vi "Autonomous Independent.vi"() -> ()   [LabVIEW 2016]
doc: "This VI is called when autonomous begins, and will automatically be terminated when autonomous ends. You can carry out timed or sensor driven robot movement independently without needing to return to the caller."
uses:
  <vilib>/Rock Robotics/Network Tables/NT Read String.vi
  Robot Global Data.vi
  <vilib>/Rock Robotics/WPI/Utilities/WPI_GetSetVariantRefNum.vi
  <vilib>/Rock Robotics/Network Tables/NT Write Numeric Array.vi
  2039lib.lvlib
panel:
  out "Doing Something":bool=TRUE
  # "Be sure to right-click and choose Data Operations>>Make Current Value default if you want to save the array values with the VI"
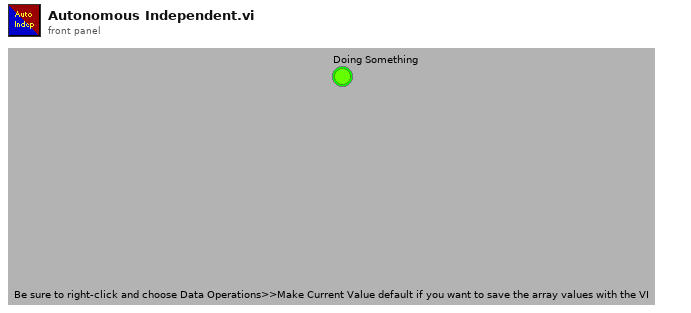
[diagram p1: front panel]
types:
  T1 = typedef "WPI_RobotDriveDevRef.ctl" = cluster{"DevStatus":errorcluster, "Motors[]":T2[], "Square Inputs":bool, "Max Output":dbl}
  T2 = typedef "WPI_MotorControlDeviceRef.ctl" = cluster{"DeviceStatus":errorcluster, "Type":T3, "PWM":cluster{"PWM Channel":T4, "DeadBand":T5}, "CAN":cluster{"Device Number":u8, "SetOutput VI Ref":variant, "GetOutput VI Ref":variant, "Enable VI Ref":variant, "Disable VI Ref":variant, "Data":variant}, "Invert":bool}
  T3 = typedef "WPI_MotorControlType.ctl" = enum16{"PWM", "CAN"}
  T4 = typedef "FPGA_DIOPWMChannel.ctl" = enum8{"PWM 0", "PWM 1", "PWM 2", "PWM 3", "PWM 4", "PWM 5", "PWM 6", "PWM 7", "PWM 8", "PWM 9", "PWM MXP 0", "PWM MXP 1", "PWM MXP 2", "PWM MXP 3", "PWM MXP 4", "PWM MXP 5", "PWM MXP 6", "PWM MXP 7", "PWM MXP 8", "PWM MXP 9", "Invalid"}
  T5 = typedef "WPI_PWMDeadband.ctl" = cluster{"Name":string, "maxPositivePwm":i32, "minPositivePwm":i32, "centerPwm":i32, "maxNegativePwm":i32, "minNegativePwm":i32, "angularRange":u16}
  T6 = typedef "WPI_ServoDeviceRef.ctl" = cluster{"DeviceStatus":errorcluster, "PWM Channel":T4, "DeadBand":T5}
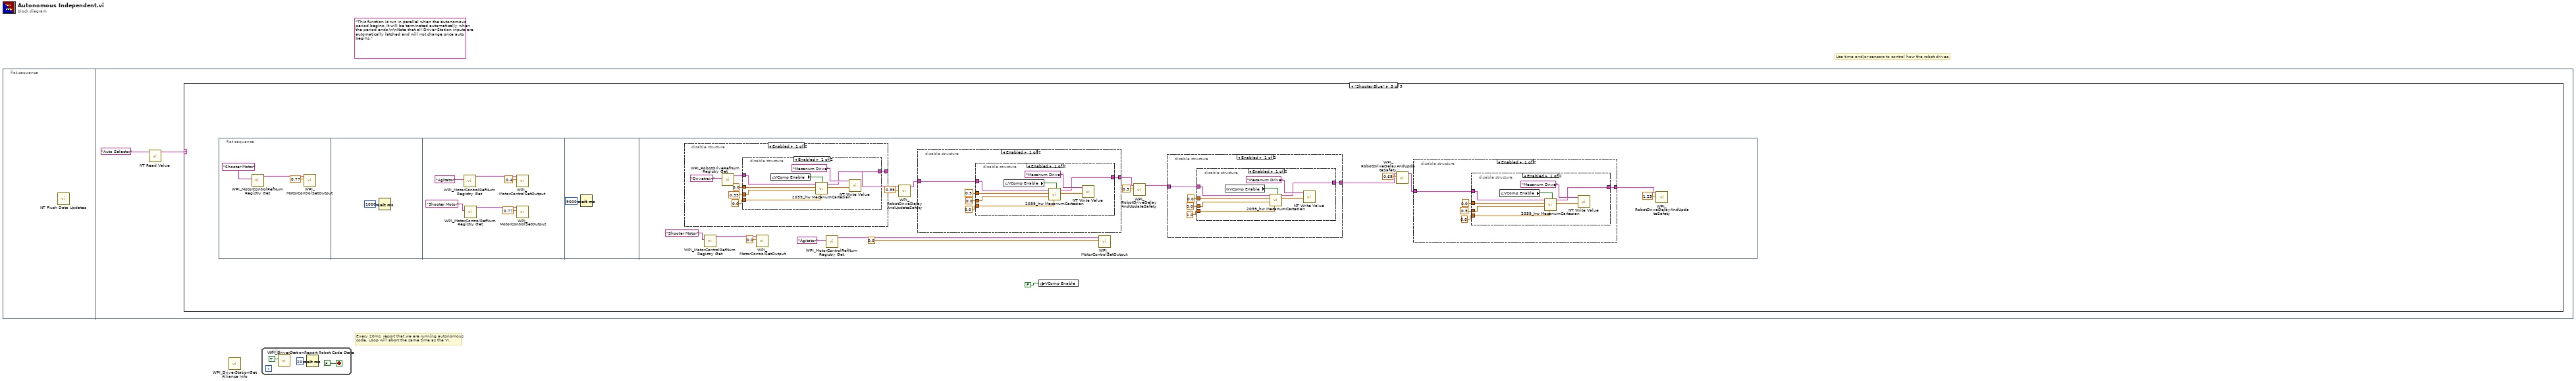
[diagram p0: block diagram]
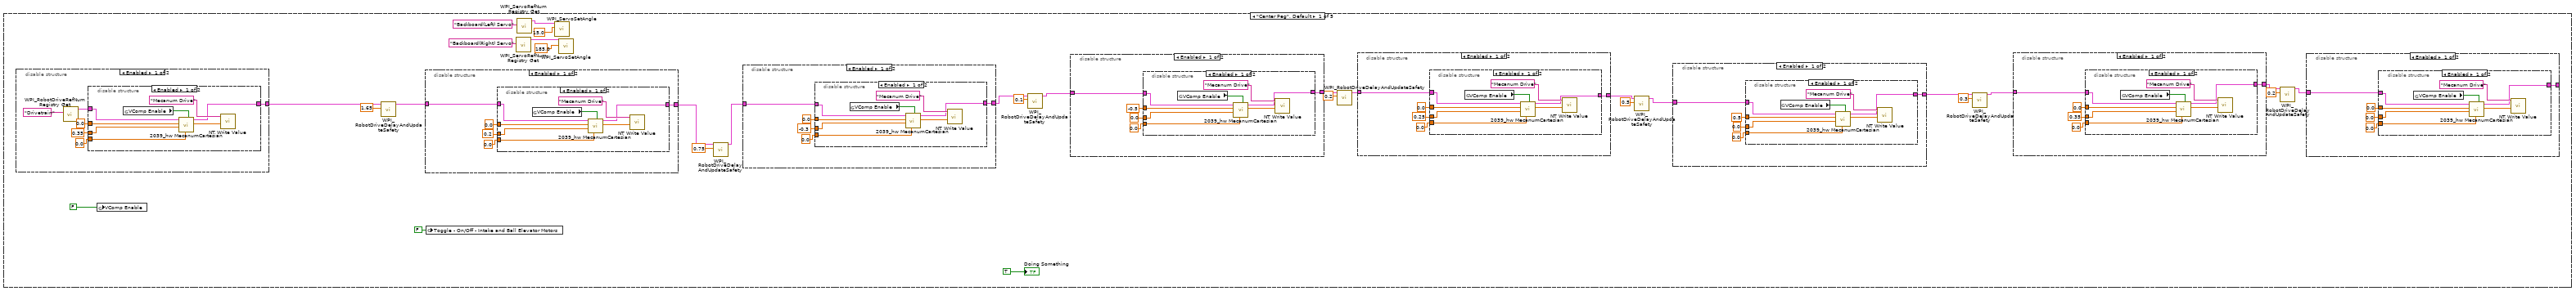
[diagram p2: hidden frame]
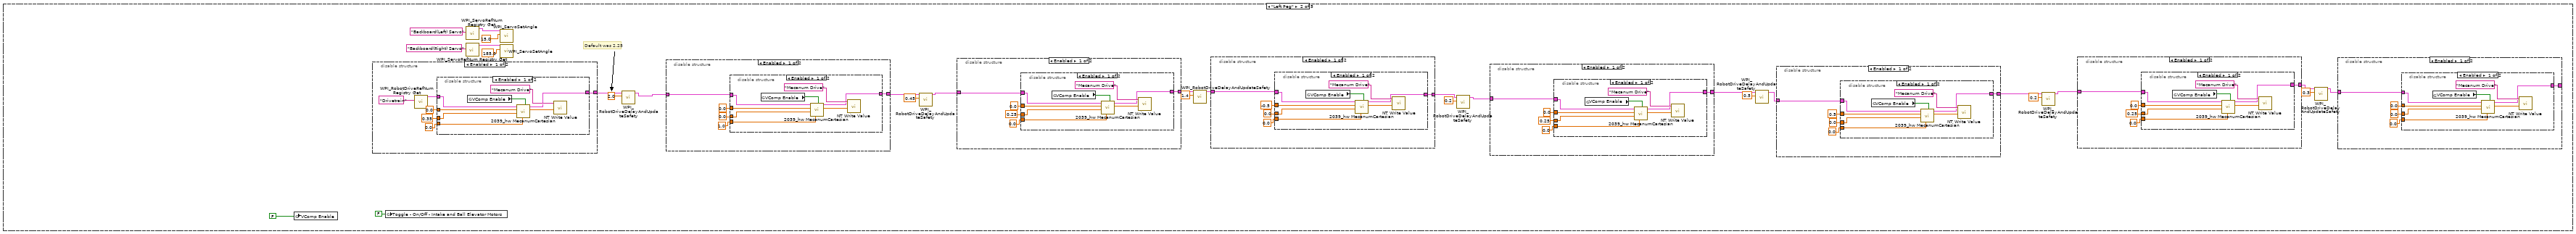
[diagram p19: hidden frame]
diagram:
  (unwired) "This function is run in parallel when the autonomous period begins. It will be terminated automatically when the period ends.\n\nNote that all Driver Station inputs are automatically latched and will not change once auto begins."
  # "Every 20ms, report that we are running autonomous\ncode. Loop will abort the same time as the VI."
  # "Use time and/or sensors to control how the robot drives."
  n1 = flat-sequence {
    frame #0 {
      n2 = call <vilib>:"NT Flush Data Updates.vi"() -> ()  [unwired: 11 in, 1 out]
    }
    frame #1 {
      n3 = call-poly <vilib>:"NT Read Value.vi"("Name"="Auto Selector") -> ("String"=w1:string)  [unwired: 9 in, 1 out]
      n4 = case shown="\"Shooter Blue\"" w1 {
        frame "Center Peg", Default {
          n5 = disable-structure shown="Enabled" {
            disable-tunnel: [w124 _] -> w31
            frame Enabled {
              n6 = call <vilib>:"WPI_RobotDriveRefNum Registry Get.vi"("refnum name"="Drivetrain") -> ("RobotDriveDevRef"=w128:T1)  [unwired: 1 in, 9 out]
              n7 = disable-structure shown="Enabled" {
                disable-tunnel: w128 -> [w137 _]
                disable-tunnel: 0.0 -> [w136 _]
                disable-tunnel: 0.0 -> [w133 _]
                disable-tunnel: 0.35 -> [w132 _]
                disable-tunnel: [w130 _] -> w124
                frame Enabled {
                  n8 = global read "Robot Global Data.vi" "VComp Enable"() -> (w131:bool)
                  n9 = call "2039_hw MecanumCartesian.vi"("VComp Scaling"=w131, "Rotation"=w136, "Y"=w132, "X"=w133, "RobotDriveDevRef"=w137) -> ("Motor Values"=w134:dbl[], "RobotDriveDevRef"=w130:T1)  [unwired: 4 in, 1 out]
                  n10 = call-poly <vilib>:"NT Write Value.vi"("Numeric Array"=w134, "Name"="Mecanum Drive") -> ()  [unwired: 9 in, 1 out]
                }
                frame Disabled {
                }
              }
            }
            frame Disabled {
            }
          }
          n11 = global write "Robot Global Data.vi" "VComp Enable"(FALSE) -> ()
          n12 = call <vilib>:"WPI_RobotDriveDelayAndUpdateSafety.vi"("Delay (s)"=1.65, "RobotDriveDevRef"=w31) -> ("RobotDriveDevRef 2"=w5:T1)  [unwired: 8 in, 1 out]
          n13 = disable-structure shown="Enabled" {
            disable-tunnel: [w34 _] -> w7
            disable-tunnel: w5 -> [w33 _]
            frame Enabled {
              n14 = disable-structure shown="Enabled" {
                disable-tunnel: 0.0 -> [w45 _]
                disable-tunnel: 0.0 -> [w42 _]
                disable-tunnel: 0.2 -> [w41 _]
                disable-tunnel: [w39 _] -> w34
                disable-tunnel: w33 -> [w38 _]
                frame Enabled {
                  n15 = global read "Robot Global Data.vi" "VComp Enable"() -> (w40:bool)
                  n16 = call "2039_hw MecanumCartesian.vi"("VComp Scaling"=w40, "Rotation"=w45, "Y"=w41, "X"=w42, "RobotDriveDevRef"=w38) -> ("Motor Values"=w43:dbl[], "RobotDriveDevRef"=w39:T1)  [unwired: 4 in, 1 out]
                  n17 = call-poly <vilib>:"NT Write Value.vi"("Numeric Array"=w43, "Name"="Mecanum Drive") -> ()  [unwired: 9 in, 1 out]
                }
                frame Disabled {
                }
              }
            }
            frame Disabled {
            }
          }
          n18 = global write "Robot Global Data.vi" "Toggle - On/Off - Intake and Ball Elevator Motors"(FALSE ("Toggle - On/Off - Intake and Ball Elevator Motors")) -> ()
          n19 = call <vilib>:"WPI_ServoRefNum Registry Get.vi"("refnum name"="Backboard(Right) Servo") -> ("ServoDeviceRef"=w17:T6)  [unwired: 9 in, 1 out]
          n20 = call <vilib>:"WPI_ServoRefNum Registry Get.vi"("refnum name"="Backboard(Left) Servo") -> ("ServoDeviceRef"=w18:T6)  [unwired: 9 in, 1 out]
          n21 = call <vilib>:"WPI_ServoSetAngle.vi"("Angle"=15.0 ("f"), "ServoDeviceRef"=w18) -> ()  [unwired: 8 in, 2 out]
          n22 = call <vilib>:"WPI_ServoSetAngle.vi"("Angle"=185.0 ("f"), "ServoDeviceRef"=w17) -> ()  [unwired: 8 in, 2 out]
          n23 = call <vilib>:"WPI_RobotDriveDelayAndUpdateSafety.vi"("Delay (s)"=0.75, "RobotDriveDevRef"=w7) -> ("RobotDriveDevRef 2"=w4:T1)  [unwired: 8 in, 1 out]
          n24 = disable-structure shown="Enabled" {
            disable-tunnel: w4 -> [w47 _]
            disable-tunnel: [w46 _] -> w11
            frame Enabled {
              n25 = disable-structure shown="Enabled" {
                disable-tunnel: w47 -> [w58 _]
                disable-tunnel: 0.0 -> [w57 _]
                disable-tunnel: 0.0 -> [w54 _]
                disable-tunnel: -0.3 -> [w53 _]
                disable-tunnel: [w51 _] -> w46
                frame Enabled {
                  n26 = global read "Robot Global Data.vi" "VComp Enable"() -> (w52:bool)
                  n27 = call "2039_hw MecanumCartesian.vi"("VComp Scaling"=w52, "Rotation"=w57, "Y"=w53, "X"=w54, "RobotDriveDevRef"=w58) -> ("Motor Values"=w55:dbl[], "RobotDriveDevRef"=w51:T1)  [unwired: 4 in, 1 out]
                  n28 = call-poly <vilib>:"NT Write Value.vi"("Numeric Array"=w55, "Name"="Mecanum Drive") -> ()  [unwired: 9 in, 1 out]
                }
                frame Disabled {
                }
              }
            }
            frame Disabled {
            }
          }
          n29 = call <vilib>:"WPI_RobotDriveDelayAndUpdateSafety.vi"("Delay (s)"=0.1, "RobotDriveDevRef"=w11) -> ("RobotDriveDevRef 2"=w10:T1)  [unwired: 8 in, 1 out]
          n30 = disable-structure shown="Enabled" {
            disable-tunnel: w10 -> [w112 _]
            disable-tunnel: [w111 _] -> w29
            frame Enabled {
              n31 = disable-structure shown="Enabled" {
                disable-tunnel: w112 -> [w123 _]
                disable-tunnel: 0.0 -> [w122 _]
                disable-tunnel: -0.5 -> [w119 _]
                disable-tunnel: 0.0 -> [w118 _]
                disable-tunnel: [w116 _] -> w111
                frame Enabled {
                  n32 = global read "Robot Global Data.vi" "VComp Enable"() -> (w117:bool)
                  n33 = call "2039_hw MecanumCartesian.vi"("VComp Scaling"=w117, "Rotation"=w122, "Y"=w118, "X"=w119, "RobotDriveDevRef"=w123) -> ("Motor Values"=w120:dbl[], "RobotDriveDevRef"=w116:T1)  [unwired: 4 in, 1 out]
                  n34 = call-poly <vilib>:"NT Write Value.vi"("Numeric Array"=w120, "Name"="Mecanum Drive") -> ()  [unwired: 9 in, 1 out]
                }
                frame Disabled {
                }
              }
            }
            frame Disabled {
            }
          }
          n35 = call <vilib>:"WPI_RobotDriveDelayAndUpdateSafety.vi"("Delay (s)"=0.2, "RobotDriveDevRef"=w29) -> ("RobotDriveDevRef 2"=w28:T1)  [unwired: 8 in, 1 out]
          n36 = disable-structure shown="Enabled" {
            disable-tunnel: w28 -> [w99 _]
            disable-tunnel: [w98 _] -> w26
            frame Enabled {
              n37 = disable-structure shown="Enabled" {
                disable-tunnel: w99 -> [w110 _]
                disable-tunnel: 0.0 -> [w109 _]
                disable-tunnel: 0.0 -> [w106 _]
                disable-tunnel: 0.25 -> [w105 _]
                disable-tunnel: [w103 _] -> w98
                frame Enabled {
                  n38 = global read "Robot Global Data.vi" "VComp Enable"() -> (w104:bool)
                  n39 = call "2039_hw MecanumCartesian.vi"("VComp Scaling"=w104, "Rotation"=w109, "Y"=w105, "X"=w106, "RobotDriveDevRef"=w110) -> ("Motor Values"=w107:dbl[], "RobotDriveDevRef"=w103:T1)  [unwired: 4 in, 1 out]
                  n40 = call-poly <vilib>:"NT Write Value.vi"("Numeric Array"=w107, "Name"="Mecanum Drive") -> ()  [unwired: 9 in, 1 out]
                }
                frame Disabled {
                }
              }
            }
            frame Disabled {
            }
          }
          n41 = call <vilib>:"WPI_RobotDriveDelayAndUpdateSafety.vi"("Delay (s)"=0.5, "RobotDriveDevRef"=w26) -> ("RobotDriveDevRef 2"=w25:T1)  [unwired: 8 in, 1 out]
          n42 = disable-structure shown="Enabled" {
            disable-tunnel: w25 -> [w86 _]
            disable-tunnel: [w85 _] -> w23
            frame Enabled {
              n43 = disable-structure shown="Enabled" {
                disable-tunnel: w86 -> [w97 _]
                disable-tunnel: 0.0 -> [w96 _]
                disable-tunnel: 0.5 -> [w93 _]
                disable-tunnel: 0.0 -> [w92 _]
                disable-tunnel: [w90 _] -> w85
                frame Enabled {
                  n44 = global read "Robot Global Data.vi" "VComp Enable"() -> (w91:bool)
                  n45 = call "2039_hw MecanumCartesian.vi"("VComp Scaling"=w91, "Rotation"=w96, "Y"=w92, "X"=w93, "RobotDriveDevRef"=w97) -> ("Motor Values"=w94:dbl[], "RobotDriveDevRef"=w90:T1)  [unwired: 4 in, 1 out]
                  n46 = call-poly <vilib>:"NT Write Value.vi"("Numeric Array"=w94, "Name"="Mecanum Drive") -> ()  [unwired: 9 in, 1 out]
                }
                frame Disabled {
                }
              }
            }
            frame Disabled {
            }
          }
          n47 = call <vilib>:"WPI_RobotDriveDelayAndUpdateSafety.vi"("Delay (s)"=0.3, "RobotDriveDevRef"=w23) -> ("RobotDriveDevRef 2"=w21:T1)  [unwired: 8 in, 1 out]
          n48 = disable-structure shown="Enabled" {
            disable-tunnel: w21 -> [w73 _]
            disable-tunnel: [w72 _] -> w14
            frame Enabled {
              n49 = disable-structure shown="Enabled" {
                disable-tunnel: w73 -> [w84 _]
                disable-tunnel: 0.0 -> [w83 _]
                disable-tunnel: 0.0 -> [w80 _]
                disable-tunnel: 0.35 -> [w79 _]
                disable-tunnel: [w77 _] -> w72
                frame Enabled {
                  n50 = global read "Robot Global Data.vi" "VComp Enable"() -> (w78:bool)
                  n51 = call "2039_hw MecanumCartesian.vi"("VComp Scaling"=w78, "Rotation"=w83, "Y"=w79, "X"=w80, "RobotDriveDevRef"=w84) -> ("Motor Values"=w81:dbl[], "RobotDriveDevRef"=w77:T1)  [unwired: 4 in, 1 out]
                  n52 = call-poly <vilib>:"NT Write Value.vi"("Numeric Array"=w81, "Name"="Mecanum Drive") -> ()  [unwired: 9 in, 1 out]
                }
                frame Disabled {
                }
              }
            }
            frame Disabled {
            }
          }
          n53 = call <vilib>:"WPI_RobotDriveDelayAndUpdateSafety.vi"("Delay (s)"=0.2, "RobotDriveDevRef"=w14) -> ("RobotDriveDevRef 2"=w13:T1)  [unwired: 8 in, 1 out]
          n54 = disable-structure shown="Enabled" {
            disable-tunnel: w13 -> [w60 _]
            disable-tunnel: [w59 _] -> _
            frame Enabled {
              n55 = disable-structure shown="Enabled" {
                disable-tunnel: w60 -> [w71 _]
                disable-tunnel: 0.0 -> [w70 _]
                disable-tunnel: 0.0 -> [w67 _]
                disable-tunnel: 0.0 -> [w66 _]
                disable-tunnel: [w64 _] -> w59
                frame Enabled {
                  n56 = global read "Robot Global Data.vi" "VComp Enable"() -> (w65:bool)
                  n57 = call "2039_hw MecanumCartesian.vi"("VComp Scaling"=w65, "Rotation"=w70, "Y"=w66, "X"=w67, "RobotDriveDevRef"=w71) -> ("Motor Values"=w68:dbl[], "RobotDriveDevRef"=w64:T1)  [unwired: 4 in, 1 out]
                  n58 = call-poly <vilib>:"NT Write Value.vi"("Numeric Array"=w68, "Name"="Mecanum Drive") -> ()  [unwired: 9 in, 1 out]
                }
                frame Disabled {
                }
              }
            }
            frame Disabled {
            }
          }
          "Doing Something" <- TRUE
        }
        frame "Left Peg" {
          # "Default was 2.25"
          n59 = global write "Robot Global Data.vi" "VComp Enable"(FALSE) -> ()
          n60 = disable-structure shown="Enabled" {
            disable-tunnel: [w258 _] -> w166
            frame Enabled {
              n61 = call <vilib>:"WPI_RobotDriveRefNum Registry Get.vi"("refnum name"="Drivetrain") -> ("RobotDriveDevRef"=w262:T1)  [unwired: 1 in, 9 out]
              n62 = disable-structure shown="Enabled" {
                disable-tunnel: w262 -> [w271 _]
                disable-tunnel: 0.0 -> [w270 _]
                disable-tunnel: 0.0 -> [w267 _]
                disable-tunnel: 0.35 -> [w266 _]
                disable-tunnel: [w264 _] -> w258
                frame Enabled {
                  n63 = global read "Robot Global Data.vi" "VComp Enable"() -> (w265:bool)
                  n64 = call "2039_hw MecanumCartesian.vi"("VComp Scaling"=w265, "Rotation"=w270, "Y"=w266, "X"=w267, "RobotDriveDevRef"=w271) -> ("Motor Values"=w268:dbl[], "RobotDriveDevRef"=w264:T1)  [unwired: 4 in, 1 out]
                  n65 = call-poly <vilib>:"NT Write Value.vi"("Numeric Array"=w268, "Name"="Mecanum Drive") -> ()  [unwired: 9 in, 1 out]
                }
                frame Disabled {
                }
              }
            }
            frame Disabled {
            }
          }
          n66 = global write "Robot Global Data.vi" "Toggle - On/Off - Intake and Ball Elevator Motors"(FALSE ("Toggle - On/Off - Intake and Ball Elevator Motors")) -> ()
          n67 = call <vilib>:"WPI_ServoRefNum Registry Get.vi"("refnum name"="Backboard(Right) Servo") -> ("ServoDeviceRef"=w153:T6)  [unwired: 9 in, 1 out]
          n68 = call <vilib>:"WPI_ServoRefNum Registry Get.vi"("refnum name"="Backboard(Left) Servo") -> ("ServoDeviceRef"=w154:T6)  [unwired: 9 in, 1 out]
          n69 = call <vilib>:"WPI_ServoSetAngle.vi"("Angle"=15.0 ("f"), "ServoDeviceRef"=w154) -> ()  [unwired: 8 in, 2 out]
          n70 = call <vilib>:"WPI_ServoSetAngle.vi"("Angle"=185.0 ("f"), "ServoDeviceRef"=w153) -> ()  [unwired: 8 in, 2 out]
          n71 = call <vilib>:"WPI_RobotDriveDelayAndUpdateSafety.vi"("Delay (s)"=2.0, "RobotDriveDevRef"=w166) -> ("RobotDriveDevRef 2"=w146:T1)  [unwired: 8 in, 1 out]
          n72 = disable-structure shown="Enabled" {
            disable-tunnel: w146 -> [w168 _]
            disable-tunnel: [w167 _] -> w140
            frame Enabled {
              n73 = disable-structure shown="Enabled" {
                disable-tunnel: w168 -> [w179 _]
                disable-tunnel: 1.0 -> [w178 _]
                disable-tunnel: 0.0 -> [w175 _]
                disable-tunnel: 0.0 -> [w174 _]
                disable-tunnel: [w172 _] -> w167
                frame Enabled {
                  n74 = global read "Robot Global Data.vi" "VComp Enable"() -> (w173:bool)
                  n75 = call "2039_hw MecanumCartesian.vi"("VComp Scaling"=w173, "Rotation"=w178, "Y"=w174, "X"=w175, "RobotDriveDevRef"=w179) -> ("Motor Values"=w176:dbl[], "RobotDriveDevRef"=w172:T1)  [unwired: 4 in, 1 out]
                  n76 = call-poly <vilib>:"NT Write Value.vi"("Numeric Array"=w176, "Name"="Mecanum Drive") -> ()  [unwired: 9 in, 1 out]
                }
                frame Disabled {
                }
              }
            }
            frame Disabled {
            }
          }
          n77 = call <vilib>:"WPI_RobotDriveDelayAndUpdateSafety.vi"("Delay (s)"=0.45, "RobotDriveDevRef"=w140) -> ("RobotDriveDevRef 2"=w147:T1)  [unwired: 8 in, 1 out]
          n78 = disable-structure shown="Enabled" {
            disable-tunnel: w147 -> [w246 _]
            disable-tunnel: [w245 _] -> w164
            frame Enabled {
              n79 = disable-structure shown="Enabled" {
                disable-tunnel: w246 -> [w257 _]
                disable-tunnel: 0.0 -> [w256 _]
                disable-tunnel: 0.0 -> [w253 _]
                disable-tunnel: 0.25 -> [w252 _]
                disable-tunnel: [w250 _] -> w245
                frame Enabled {
                  n80 = global read "Robot Global Data.vi" "VComp Enable"() -> (w251:bool)
                  n81 = call "2039_hw MecanumCartesian.vi"("VComp Scaling"=w251, "Rotation"=w256, "Y"=w252, "X"=w253, "RobotDriveDevRef"=w257) -> ("Motor Values"=w254:dbl[], "RobotDriveDevRef"=w250:T1)  [unwired: 4 in, 1 out]
                  n82 = call-poly <vilib>:"NT Write Value.vi"("Numeric Array"=w254, "Name"="Mecanum Drive") -> ()  [unwired: 9 in, 1 out]
                }
                frame Disabled {
                }
              }
            }
            frame Disabled {
            }
          }
          n83 = call <vilib>:"WPI_RobotDriveDelayAndUpdateSafety.vi"("Delay (s)"=1.4, "RobotDriveDevRef"=w164) -> ("RobotDriveDevRef 2"=w163:T1)  [unwired: 8 in, 1 out]
          n84 = disable-structure shown="Enabled" {
            disable-tunnel: w163 -> [w233 _]
            disable-tunnel: [w232 _] -> w161
            frame Enabled {
              n85 = disable-structure shown="Enabled" {
                disable-tunnel: w233 -> [w244 _]
                disable-tunnel: 0.0 -> [w243 _]
                disable-tunnel: -0.5 -> [w240 _]
                disable-tunnel: 0.0 -> [w239 _]
                disable-tunnel: [w237 _] -> w232
                frame Enabled {
                  n86 = global read "Robot Global Data.vi" "VComp Enable"() -> (w238:bool)
                  n87 = call "2039_hw MecanumCartesian.vi"("VComp Scaling"=w238, "Rotation"=w243, "Y"=w239, "X"=w240, "RobotDriveDevRef"=w244) -> ("Motor Values"=w241:dbl[], "RobotDriveDevRef"=w237:T1)  [unwired: 4 in, 1 out]
                  n88 = call-poly <vilib>:"NT Write Value.vi"("Numeric Array"=w241, "Name"="Mecanum Drive") -> ()  [unwired: 9 in, 1 out]
                }
                frame Disabled {
                }
              }
            }
            frame Disabled {
            }
          }
          n89 = call <vilib>:"WPI_RobotDriveDelayAndUpdateSafety.vi"("Delay (s)"=0.2, "RobotDriveDevRef"=w161) -> ("RobotDriveDevRef 2"=w141:T1)  [unwired: 8 in, 1 out]
          n90 = disable-structure shown="Enabled" {
            disable-tunnel: w141 -> [w181 _]
            disable-tunnel: [w180 _] -> w144
            frame Enabled {
              n91 = disable-structure shown="Enabled" {
                disable-tunnel: w181 -> [w192 _]
                disable-tunnel: 0.0 -> [w191 _]
                disable-tunnel: 0.0 -> [w188 _]
                disable-tunnel: 0.25 -> [w187 _]
                disable-tunnel: [w185 _] -> w180
                frame Enabled {
                  n92 = global read "Robot Global Data.vi" "VComp Enable"() -> (w186:bool)
                  n93 = call "2039_hw MecanumCartesian.vi"("VComp Scaling"=w186, "Rotation"=w191, "Y"=w187, "X"=w188, "RobotDriveDevRef"=w192) -> ("Motor Values"=w189:dbl[], "RobotDriveDevRef"=w185:T1)  [unwired: 4 in, 1 out]
                  n94 = call-poly <vilib>:"NT Write Value.vi"("Numeric Array"=w189, "Name"="Mecanum Drive") -> ()  [unwired: 9 in, 1 out]
                }
                frame Disabled {
                }
              }
            }
            frame Disabled {
            }
          }
          n95 = call <vilib>:"WPI_RobotDriveDelayAndUpdateSafety.vi"("Delay (s)"=0.5, "RobotDriveDevRef"=w144) -> ("RobotDriveDevRef 2"=w142:T1)  [unwired: 8 in, 1 out]
          n96 = disable-structure shown="Enabled" {
            disable-tunnel: w142 -> [w220 _]
            disable-tunnel: [w219 _] -> w159
            frame Enabled {
              n97 = disable-structure shown="Enabled" {
                disable-tunnel: w220 -> [w231 _]
                disable-tunnel: 0.0 -> [w230 _]
                disable-tunnel: 0.5 -> [w227 _]
                disable-tunnel: 0.0 -> [w226 _]
                disable-tunnel: [w224 _] -> w219
                frame Enabled {
                  n98 = global read "Robot Global Data.vi" "VComp Enable"() -> (w225:bool)
                  n99 = call "2039_hw MecanumCartesian.vi"("VComp Scaling"=w225, "Rotation"=w230, "Y"=w226, "X"=w227, "RobotDriveDevRef"=w231) -> ("Motor Values"=w228:dbl[], "RobotDriveDevRef"=w224:T1)  [unwired: 4 in, 1 out]
                  n100 = call-poly <vilib>:"NT Write Value.vi"("Numeric Array"=w228, "Name"="Mecanum Drive") -> ()  [unwired: 9 in, 1 out]
                }
                frame Disabled {
                }
              }
            }
            frame Disabled {
            }
          }
          n101 = call <vilib>:"WPI_RobotDriveDelayAndUpdateSafety.vi"("Delay (s)"=0.2, "RobotDriveDevRef"=w159) -> ("RobotDriveDevRef 2"=w157:T1)  [unwired: 8 in, 1 out]
          n102 = disable-structure shown="Enabled" {
            disable-tunnel: w157 -> [w207 _]
            disable-tunnel: [w206 _] -> w150
            frame Enabled {
              n103 = disable-structure shown="Enabled" {
                disable-tunnel: w207 -> [w218 _]
                disable-tunnel: 0.0 -> [w217 _]
                disable-tunnel: 0.0 -> [w214 _]
                disable-tunnel: 0.25 -> [w213 _]
                disable-tunnel: [w211 _] -> w206
                frame Enabled {
                  n104 = global read "Robot Global Data.vi" "VComp Enable"() -> (w212:bool)
                  n105 = call "2039_hw MecanumCartesian.vi"("VComp Scaling"=w212, "Rotation"=w217, "Y"=w213, "X"=w214, "RobotDriveDevRef"=w218) -> ("Motor Values"=w215:dbl[], "RobotDriveDevRef"=w211:T1)  [unwired: 4 in, 1 out]
                  n106 = call-poly <vilib>:"NT Write Value.vi"("Numeric Array"=w215, "Name"="Mecanum Drive") -> ()  [unwired: 9 in, 1 out]
                }
                frame Disabled {
                }
              }
            }
            frame Disabled {
            }
          }
          n107 = call <vilib>:"WPI_RobotDriveDelayAndUpdateSafety.vi"("Delay (s)"=0.3, "RobotDriveDevRef"=w150) -> ("RobotDriveDevRef 2"=w149:T1)  [unwired: 8 in, 1 out]
          n108 = disable-structure shown="Enabled" {
            disable-tunnel: w149 -> [w194 _]
            disable-tunnel: [w193 _] -> _
            frame Enabled {
              n109 = disable-structure shown="Enabled" {
                disable-tunnel: w194 -> [w205 _]
                disable-tunnel: 0.0 -> [w204 _]
                disable-tunnel: 0.0 -> [w201 _]
                disable-tunnel: 0.0 -> [w200 _]
                disable-tunnel: [w198 _] -> w193
                frame Enabled {
                  n110 = global read "Robot Global Data.vi" "VComp Enable"() -> (w199:bool)
                  n111 = call "2039_hw MecanumCartesian.vi"("VComp Scaling"=w199, "Rotation"=w204, "Y"=w200, "X"=w201, "RobotDriveDevRef"=w205) -> ("Motor Values"=w202:dbl[], "RobotDriveDevRef"=w198:T1)  [unwired: 4 in, 1 out]
                  n112 = call-poly <vilib>:"NT Write Value.vi"("Numeric Array"=w202, "Name"="Mecanum Drive") -> ()  [unwired: 9 in, 1 out]
                }
                frame Disabled {
                }
              }
            }
            frame Disabled {
            }
          }
        }
        frame "Right Peg" {
          # "Default was 2.25"
          n113 = global write "Robot Global Data.vi" "VComp Enable"(FALSE) -> ()
          n114 = disable-structure shown="Enabled" {
            disable-tunnel: [w392 _] -> w300
            frame Enabled {
              n115 = call <vilib>:"WPI_RobotDriveRefNum Registry Get.vi"("refnum name"="Drivetrain") -> ("RobotDriveDevRef"=w396:T1)  [unwired: 1 in, 9 out]
              n116 = disable-structure shown="Enabled" {
                disable-tunnel: w396 -> [w405 _]
                disable-tunnel: 0.0 -> [w404 _]
                disable-tunnel: 0.0 -> [w401 _]
                disable-tunnel: 0.35 -> [w400 _]
                disable-tunnel: [w398 _] -> w392
                frame Enabled {
                  n117 = global read "Robot Global Data.vi" "VComp Enable"() -> (w399:bool)
                  n118 = call "2039_hw MecanumCartesian.vi"("VComp Scaling"=w399, "Rotation"=w404, "Y"=w400, "X"=w401, "RobotDriveDevRef"=w405) -> ("Motor Values"=w402:dbl[], "RobotDriveDevRef"=w398:T1)  [unwired: 4 in, 1 out]
                  n119 = call-poly <vilib>:"NT Write Value.vi"("Numeric Array"=w402, "Name"="Mecanum Drive") -> ()  [unwired: 9 in, 1 out]
                }
                frame Disabled {
                }
              }
            }
            frame Disabled {
            }
          }
          n120 = global write "Robot Global Data.vi" "Toggle - On/Off - Intake and Ball Elevator Motors"(FALSE ("Toggle - On/Off - Intake and Ball Elevator Motors")) -> ()
          n121 = call <vilib>:"WPI_ServoRefNum Registry Get.vi"("refnum name"="Backboard(Right) Servo") -> ("ServoDeviceRef"=w287:T6)  [unwired: 9 in, 1 out]
          n122 = call <vilib>:"WPI_ServoRefNum Registry Get.vi"("refnum name"="Backboard(Left) Servo") -> ("ServoDeviceRef"=w288:T6)  [unwired: 9 in, 1 out]
          n123 = call <vilib>:"WPI_ServoSetAngle.vi"("Angle"=15.0 ("f"), "ServoDeviceRef"=w288) -> ()  [unwired: 8 in, 2 out]
          n124 = call <vilib>:"WPI_ServoSetAngle.vi"("Angle"=185.0 ("f"), "ServoDeviceRef"=w287) -> ()  [unwired: 8 in, 2 out]
          n125 = call <vilib>:"WPI_RobotDriveDelayAndUpdateSafety.vi"("Delay (s)"=2.0, "RobotDriveDevRef"=w300) -> ("RobotDriveDevRef 2"=w280:T1)  [unwired: 8 in, 1 out]
          n126 = disable-structure shown="Enabled" {
            disable-tunnel: w280 -> [w302 _]
            disable-tunnel: [w301 _] -> w274
            frame Enabled {
              n127 = disable-structure shown="Enabled" {
                disable-tunnel: w302 -> [w313 _]
                disable-tunnel: -1.0 -> [w312 _]
                disable-tunnel: 0.0 -> [w309 _]
                disable-tunnel: 0.0 -> [w308 _]
                disable-tunnel: [w306 _] -> w301
                frame Enabled {
                  n128 = global read "Robot Global Data.vi" "VComp Enable"() -> (w307:bool)
                  n129 = call "2039_hw MecanumCartesian.vi"("VComp Scaling"=w307, "Rotation"=w312, "Y"=w308, "X"=w309, "RobotDriveDevRef"=w313) -> ("Motor Values"=w310:dbl[], "RobotDriveDevRef"=w306:T1)  [unwired: 4 in, 1 out]
                  n130 = call-poly <vilib>:"NT Write Value.vi"("Numeric Array"=w310, "Name"="Mecanum Drive") -> ()  [unwired: 9 in, 1 out]
                }
                frame Disabled {
                }
              }
            }
            frame Disabled {
            }
          }
          n131 = call <vilib>:"WPI_RobotDriveDelayAndUpdateSafety.vi"("Delay (s)"=0.45, "RobotDriveDevRef"=w274) -> ("RobotDriveDevRef 2"=w281:T1)  [unwired: 8 in, 1 out]
          n132 = disable-structure shown="Enabled" {
            disable-tunnel: w281 -> [w380 _]
            disable-tunnel: [w379 _] -> w298
            frame Enabled {
              n133 = disable-structure shown="Enabled" {
                disable-tunnel: w380 -> [w391 _]
                disable-tunnel: 0.0 -> [w390 _]
                disable-tunnel: 0.0 -> [w387 _]
                disable-tunnel: 0.25 -> [w386 _]
                disable-tunnel: [w384 _] -> w379
                frame Enabled {
                  n134 = global read "Robot Global Data.vi" "VComp Enable"() -> (w385:bool)
                  n135 = call "2039_hw MecanumCartesian.vi"("VComp Scaling"=w385, "Rotation"=w390, "Y"=w386, "X"=w387, "RobotDriveDevRef"=w391) -> ("Motor Values"=w388:dbl[], "RobotDriveDevRef"=w384:T1)  [unwired: 4 in, 1 out]
                  n136 = call-poly <vilib>:"NT Write Value.vi"("Numeric Array"=w388, "Name"="Mecanum Drive") -> ()  [unwired: 9 in, 1 out]
                }
                frame Disabled {
                }
              }
            }
            frame Disabled {
            }
          }
          n137 = call <vilib>:"WPI_RobotDriveDelayAndUpdateSafety.vi"("Delay (s)"=1.4, "RobotDriveDevRef"=w298) -> ("RobotDriveDevRef 2"=w297:T1)  [unwired: 8 in, 1 out]
          n138 = disable-structure shown="Enabled" {
            disable-tunnel: w297 -> [w367 _]
            disable-tunnel: [w366 _] -> w295
            frame Enabled {
              n139 = disable-structure shown="Enabled" {
                disable-tunnel: w367 -> [w378 _]
                disable-tunnel: 0.0 -> [w377 _]
                disable-tunnel: -0.5 -> [w374 _]
                disable-tunnel: 0.0 -> [w373 _]
                disable-tunnel: [w371 _] -> w366
                frame Enabled {
                  n140 = global read "Robot Global Data.vi" "VComp Enable"() -> (w372:bool)
                  n141 = call "2039_hw MecanumCartesian.vi"("VComp Scaling"=w372, "Rotation"=w377, "Y"=w373, "X"=w374, "RobotDriveDevRef"=w378) -> ("Motor Values"=w375:dbl[], "RobotDriveDevRef"=w371:T1)  [unwired: 4 in, 1 out]
                  n142 = call-poly <vilib>:"NT Write Value.vi"("Numeric Array"=w375, "Name"="Mecanum Drive") -> ()  [unwired: 9 in, 1 out]
                }
                frame Disabled {
                }
              }
            }
            frame Disabled {
            }
          }
          n143 = call <vilib>:"WPI_RobotDriveDelayAndUpdateSafety.vi"("Delay (s)"=0.2, "RobotDriveDevRef"=w295) -> ("RobotDriveDevRef 2"=w275:T1)  [unwired: 8 in, 1 out]
          n144 = disable-structure shown="Enabled" {
            disable-tunnel: w275 -> [w315 _]
            disable-tunnel: [w314 _] -> w278
            frame Enabled {
              n145 = disable-structure shown="Enabled" {
                disable-tunnel: w315 -> [w326 _]
                disable-tunnel: 0.0 -> [w325 _]
                disable-tunnel: 0.0 -> [w322 _]
                disable-tunnel: 0.25 -> [w321 _]
                disable-tunnel: [w319 _] -> w314
                frame Enabled {
                  n146 = global read "Robot Global Data.vi" "VComp Enable"() -> (w320:bool)
                  n147 = call "2039_hw MecanumCartesian.vi"("VComp Scaling"=w320, "Rotation"=w325, "Y"=w321, "X"=w322, "RobotDriveDevRef"=w326) -> ("Motor Values"=w323:dbl[], "RobotDriveDevRef"=w319:T1)  [unwired: 4 in, 1 out]
                  n148 = call-poly <vilib>:"NT Write Value.vi"("Numeric Array"=w323, "Name"="Mecanum Drive") -> ()  [unwired: 9 in, 1 out]
                }
                frame Disabled {
                }
              }
            }
            frame Disabled {
            }
          }
          n149 = call <vilib>:"WPI_RobotDriveDelayAndUpdateSafety.vi"("Delay (s)"=0.5, "RobotDriveDevRef"=w278) -> ("RobotDriveDevRef 2"=w276:T1)  [unwired: 8 in, 1 out]
          n150 = disable-structure shown="Enabled" {
            disable-tunnel: w276 -> [w354 _]
            disable-tunnel: [w353 _] -> w293
            frame Enabled {
              n151 = disable-structure shown="Enabled" {
                disable-tunnel: w354 -> [w365 _]
                disable-tunnel: 0.0 -> [w364 _]
                disable-tunnel: 0.5 -> [w361 _]
                disable-tunnel: 0.0 -> [w360 _]
                disable-tunnel: [w358 _] -> w353
                frame Enabled {
                  n152 = global read "Robot Global Data.vi" "VComp Enable"() -> (w359:bool)
                  n153 = call "2039_hw MecanumCartesian.vi"("VComp Scaling"=w359, "Rotation"=w364, "Y"=w360, "X"=w361, "RobotDriveDevRef"=w365) -> ("Motor Values"=w362:dbl[], "RobotDriveDevRef"=w358:T1)  [unwired: 4 in, 1 out]
                  n154 = call-poly <vilib>:"NT Write Value.vi"("Numeric Array"=w362, "Name"="Mecanum Drive") -> ()  [unwired: 9 in, 1 out]
                }
                frame Disabled {
                }
              }
            }
            frame Disabled {
            }
          }
          n155 = call <vilib>:"WPI_RobotDriveDelayAndUpdateSafety.vi"("Delay (s)"=0.2, "RobotDriveDevRef"=w293) -> ("RobotDriveDevRef 2"=w291:T1)  [unwired: 8 in, 1 out]
          n156 = disable-structure shown="Enabled" {
            disable-tunnel: w291 -> [w341 _]
            disable-tunnel: [w340 _] -> w284
            frame Enabled {
              n157 = disable-structure shown="Enabled" {
                disable-tunnel: w341 -> [w352 _]
                disable-tunnel: 0.0 -> [w351 _]
                disable-tunnel: 0.0 -> [w348 _]
                disable-tunnel: 0.25 -> [w347 _]
                disable-tunnel: [w345 _] -> w340
                frame Enabled {
                  n158 = global read "Robot Global Data.vi" "VComp Enable"() -> (w346:bool)
                  n159 = call "2039_hw MecanumCartesian.vi"("VComp Scaling"=w346, "Rotation"=w351, "Y"=w347, "X"=w348, "RobotDriveDevRef"=w352) -> ("Motor Values"=w349:dbl[], "RobotDriveDevRef"=w345:T1)  [unwired: 4 in, 1 out]
                  n160 = call-poly <vilib>:"NT Write Value.vi"("Numeric Array"=w349, "Name"="Mecanum Drive") -> ()  [unwired: 9 in, 1 out]
                }
                frame Disabled {
                }
              }
            }
            frame Disabled {
            }
          }
          n161 = call <vilib>:"WPI_RobotDriveDelayAndUpdateSafety.vi"("Delay (s)"=0.3, "RobotDriveDevRef"=w284) -> ("RobotDriveDevRef 2"=w283:T1)  [unwired: 8 in, 1 out]
          n162 = disable-structure shown="Enabled" {
            disable-tunnel: w283 -> [w328 _]
            disable-tunnel: [w327 _] -> _
            frame Enabled {
              n163 = disable-structure shown="Enabled" {
                disable-tunnel: w328 -> [w339 _]
                disable-tunnel: 0.0 -> [w338 _]
                disable-tunnel: 0.0 -> [w335 _]
                disable-tunnel: 0.0 -> [w334 _]
                disable-tunnel: [w332 _] -> w327
                frame Enabled {
                  n164 = global read "Robot Global Data.vi" "VComp Enable"() -> (w333:bool)
                  n165 = call "2039_hw MecanumCartesian.vi"("VComp Scaling"=w333, "Rotation"=w338, "Y"=w334, "X"=w335, "RobotDriveDevRef"=w339) -> ("Motor Values"=w336:dbl[], "RobotDriveDevRef"=w332:T1)  [unwired: 4 in, 1 out]
                  n166 = call-poly <vilib>:"NT Write Value.vi"("Numeric Array"=w336, "Name"="Mecanum Drive") -> ()  [unwired: 9 in, 1 out]
                }
                frame Disabled {
                }
              }
            }
            frame Disabled {
            }
          }
        }
        frame "Shooter Red" {
          n167 = flat-sequence {
            frame #0 {
              n168 = call <vilib>:"WPI_MotorControlRefNum Registry Get.vi"("refnum name"="Shooter Motor") -> ("MotorControlDevRef"=w408:T2)  [unwired: 9 in, 1 out]
              n169 = call <vilib>:"WPI_MotorControlSetOutput.vi"("Output"=0.77, "MotorControlDevRef"=w408) -> ()  [unwired: 7 in, 3 out]
            }
            frame #1 {
              n170 = Wait (ms)(milliseconds to wait=u32 1000) -> ()  [unwired: 1 out]
            }
            frame #2 {
              n171 = call <vilib>:"WPI_MotorControlRefNum Registry Get.vi"("refnum name"="Agitator") -> ("MotorControlDevRef"=w416:T2)  [unwired: 9 in, 1 out]
              n172 = call <vilib>:"WPI_MotorControlRefNum Registry Get.vi"("refnum name"="Shooter Motor") -> ("MotorControlDevRef"=w414:T2)  [unwired: 9 in, 1 out]
              n173 = call <vilib>:"WPI_MotorControlSetOutput.vi"("Output"=0.4, "MotorControlDevRef"=w416) -> ()  [unwired: 7 in, 3 out]
              n174 = call <vilib>:"WPI_MotorControlSetOutput.vi"("Output"=0.77, "MotorControlDevRef"=w414) -> ()  [unwired: 7 in, 3 out]
            }
            frame #3 {
              n175 = Wait (ms)(milliseconds to wait=u32 9000) -> ()  [unwired: 1 out]
            }
            frame #4 {
              n176 = disable-structure shown="Enabled" {
                disable-tunnel: [w458 _] -> w431
                frame Enabled {
                  n177 = call <vilib>:"WPI_RobotDriveRefNum Registry Get.vi"("refnum name"="Drivetrain") -> ("RobotDriveDevRef"=w462:T1)  [unwired: 1 in, 9 out]
                  n178 = disable-structure shown="Enabled" {
                    disable-tunnel: w462 -> [w471 _]
                    disable-tunnel: 0.0 -> [w470 _]
                    disable-tunnel: 0.0 -> [w467 _]
                    disable-tunnel: -0.35 -> [w466 _]
                    disable-tunnel: [w464 _] -> w458
                    frame Enabled {
                      n179 = global read "Robot Global Data.vi" "VComp Enable"() -> (w465:bool)
                      n180 = call "2039_hw MecanumCartesian.vi"("VComp Scaling"=w465, "Rotation"=w470, "Y"=w466, "X"=w467, "RobotDriveDevRef"=w471) -> ("Motor Values"=w468:dbl[], "RobotDriveDevRef"=w464:T1)  [unwired: 4 in, 1 out]
                      n181 = call-poly <vilib>:"NT Write Value.vi"("Numeric Array"=w468, "Name"="Mecanum Drive") -> ()  [unwired: 9 in, 1 out]
                    }
                    frame Disabled {
                    }
                  }
                }
                frame Disabled {
                }
              }
              n182 = call <vilib>:"WPI_MotorControlRefNum Registry Get.vi"("refnum name"="Shooter Motor") -> ("MotorControlDevRef"=w423:T2)  [unwired: 9 in, 1 out]
              n183 = call <vilib>:"WPI_MotorControlSetOutput.vi"("Output"=0.0, "MotorControlDevRef"=w423) -> ()  [unwired: 7 in, 3 out]
              n184 = call <vilib>:"WPI_MotorControlRefNum Registry Get.vi"("refnum name"="Agitator") -> ("MotorControlDevRef"=w420:T2)  [unwired: 9 in, 1 out]
              n185 = call <vilib>:"WPI_MotorControlSetOutput.vi"("Output"=0.0, "MotorControlDevRef"=w420) -> ()  [unwired: 7 in, 3 out]
              n186 = call <vilib>:"WPI_RobotDriveDelayAndUpdateSafety.vi"("Delay (s)"=0.35, "RobotDriveDevRef"=w431) -> ("RobotDriveDevRef 2"=w429:T1)  [unwired: 8 in, 1 out]
              n187 = disable-structure shown="Enabled" {
                disable-tunnel: [w446 _] -> w427
                disable-tunnel: w429 -> [w445 _]
                frame Enabled {
                  n188 = disable-structure shown="Enabled" {
                    disable-tunnel: w445 -> [w457 _]
                    disable-tunnel: 1.0 -> [w456 _]
                    disable-tunnel: 0.0 -> [w453 _]
                    disable-tunnel: 0.0 -> [w452 _]
                    disable-tunnel: [w450 _] -> w446
                    frame Enabled {
                      n189 = global read "Robot Global Data.vi" "VComp Enable"() -> (w451:bool)
                      n190 = call "2039_hw MecanumCartesian.vi"("VComp Scaling"=w451, "Rotation"=w456, "Y"=w452, "X"=w453, "RobotDriveDevRef"=w457) -> ("Motor Values"=w454:dbl[], "RobotDriveDevRef"=w450:T1)  [unwired: 4 in, 1 out]
                      n191 = call-poly <vilib>:"NT Write Value.vi"("Numeric Array"=w454, "Name"="Mecanum Drive") -> ()  [unwired: 9 in, 1 out]
                    }
                    frame Disabled {
                    }
                  }
                }
                frame Disabled {
                }
              }
              n192 = call <vilib>:"WPI_RobotDriveDelayAndUpdateSafety.vi"("Delay (s)"=1.0, "RobotDriveDevRef"=w427) -> ("RobotDriveDevRef 2"=w426:T1)  [unwired: 8 in, 1 out]
              n193 = disable-structure shown="Enabled" {
                disable-tunnel: [w433 _] -> w424
                disable-tunnel: w426 -> [w432 _]
                frame Enabled {
                  n194 = disable-structure shown="Enabled" {
                    disable-tunnel: w432 -> [w444 _]
                    disable-tunnel: 0.0 -> [w443 _]
                    disable-tunnel: 0.0 -> [w440 _]
                    disable-tunnel: 0.5 -> [w439 _]
                    disable-tunnel: [w437 _] -> w433
                    frame Enabled {
                      n195 = global read "Robot Global Data.vi" "VComp Enable"() -> (w438:bool)
                      n196 = call "2039_hw MecanumCartesian.vi"("VComp Scaling"=w438, "Rotation"=w443, "Y"=w439, "X"=w440, "RobotDriveDevRef"=w444) -> ("Motor Values"=w441:dbl[], "RobotDriveDevRef"=w437:T1)  [unwired: 4 in, 1 out]
                      n197 = call-poly <vilib>:"NT Write Value.vi"("Numeric Array"=w441, "Name"="Mecanum Drive") -> ()  [unwired: 9 in, 1 out]
                    }
                    frame Disabled {
                    }
                  }
                }
                frame Disabled {
                }
              }
              n198 = call <vilib>:"WPI_RobotDriveDelayAndUpdateSafety.vi"("Delay (s)"=1.25, "RobotDriveDevRef"=w424) -> ()  [unwired: 8 in, 2 out]
            }
          }
          n199 = global write "Robot Global Data.vi" "VComp Enable"(FALSE) -> ()
        }
        frame "Shooter Blue" {
          n200 = flat-sequence {
            frame #0 {
              n201 = call <vilib>:"WPI_MotorControlRefNum Registry Get.vi"("refnum name"="Shooter Motor") -> ("MotorControlDevRef"=w474:T2)  [unwired: 9 in, 1 out]
              n202 = call <vilib>:"WPI_MotorControlSetOutput.vi"("Output"=0.77, "MotorControlDevRef"=w474) -> ()  [unwired: 7 in, 3 out]
            }
            frame #1 {
              n203 = Wait (ms)(milliseconds to wait=u32 1000) -> ()  [unwired: 1 out]
            }
            frame #2 {
              n204 = call <vilib>:"WPI_MotorControlRefNum Registry Get.vi"("refnum name"="Agitator") -> ("MotorControlDevRef"=w482:T2)  [unwired: 9 in, 1 out]
              n205 = call <vilib>:"WPI_MotorControlRefNum Registry Get.vi"("refnum name"="Shooter Motor") -> ("MotorControlDevRef"=w480:T2)  [unwired: 9 in, 1 out]
              n206 = call <vilib>:"WPI_MotorControlSetOutput.vi"("Output"=0.4, "MotorControlDevRef"=w482) -> ()  [unwired: 7 in, 3 out]
              n207 = call <vilib>:"WPI_MotorControlSetOutput.vi"("Output"=0.77, "MotorControlDevRef"=w480) -> ()  [unwired: 7 in, 3 out]
            }
            frame #3 {
              n208 = Wait (ms)(milliseconds to wait=u32 9000) -> ()  [unwired: 1 out]
            }
            frame #4 {
              n209 = disable-structure shown="Enabled" {
                disable-tunnel: [w540 _] -> w500
                frame Enabled {
                  n210 = call <vilib>:"WPI_RobotDriveRefNum Registry Get.vi"("refnum name"="Drivetrain") -> ("RobotDriveDevRef"=w544:T1)  [unwired: 1 in, 9 out]
                  n211 = disable-structure shown="Enabled" {
                    disable-tunnel: w544 -> [w553 _]
                    disable-tunnel: 0.0 -> [w552 _]
                    disable-tunnel: 0.0 -> [w549 _]
                    disable-tunnel: 0.35 -> [w548 _]
                    disable-tunnel: [w546 _] -> w540
                    frame Enabled {
                      n212 = global read "Robot Global Data.vi" "VComp Enable"() -> (w547:bool)
                      n213 = call "2039_hw MecanumCartesian.vi"("VComp Scaling"=w547, "Rotation"=w552, "Y"=w548, "X"=w549, "RobotDriveDevRef"=w553) -> ("Motor Values"=w550:dbl[], "RobotDriveDevRef"=w546:T1)  [unwired: 4 in, 1 out]
                      n214 = call-poly <vilib>:"NT Write Value.vi"("Numeric Array"=w550, "Name"="Mecanum Drive") -> ()  [unwired: 9 in, 1 out]
                    }
                    frame Disabled {
                    }
                  }
                }
                frame Disabled {
                }
              }
              n215 = call <vilib>:"WPI_MotorControlRefNum Registry Get.vi"("refnum name"="Shooter Motor") -> ("MotorControlDevRef"=w493:T2)  [unwired: 9 in, 1 out]
              n216 = call <vilib>:"WPI_MotorControlSetOutput.vi"("Output"=0.0, "MotorControlDevRef"=w493) -> ()  [unwired: 7 in, 3 out]
              n217 = call <vilib>:"WPI_MotorControlRefNum Registry Get.vi"("refnum name"="Agitator") -> ("MotorControlDevRef"=w490:T2)  [unwired: 9 in, 1 out]
              n218 = call <vilib>:"WPI_RobotDriveDelayAndUpdateSafety.vi"("Delay (s)"=0.35, "RobotDriveDevRef"=w500) -> ("RobotDriveDevRef 2"=w487:T1)  [unwired: 8 in, 1 out]
              n219 = disable-structure shown="Enabled" {
                disable-tunnel: [w502 _] -> w485
                disable-tunnel: w487 -> [w501 _]
                frame Enabled {
                  n220 = disable-structure shown="Enabled" {
                    disable-tunnel: w501 -> [w513 _]
                    disable-tunnel: 0.0 -> [w512 _]
                    disable-tunnel: 0.5 -> [w509 _]
                    disable-tunnel: 0.0 -> [w508 _]
                    disable-tunnel: [w506 _] -> w502
                    frame Enabled {
                      n221 = global read "Robot Global Data.vi" "VComp Enable"() -> (w507:bool)
                      n222 = call "2039_hw MecanumCartesian.vi"("VComp Scaling"=w507, "Rotation"=w512, "Y"=w508, "X"=w509, "RobotDriveDevRef"=w513) -> ("Motor Values"=w510:dbl[], "RobotDriveDevRef"=w506:T1)  [unwired: 4 in, 1 out]
                      n223 = call-poly <vilib>:"NT Write Value.vi"("Numeric Array"=w510, "Name"="Mecanum Drive") -> ()  [unwired: 9 in, 1 out]
                    }
                    frame Disabled {
                    }
                  }
                }
                frame Disabled {
                }
              }
              n224 = call <vilib>:"WPI_MotorControlSetOutput.vi"("Output"=0.0, "MotorControlDevRef"=w490) -> ()  [unwired: 7 in, 3 out]
              n225 = call <vilib>:"WPI_RobotDriveDelayAndUpdateSafety.vi"("Delay (s)"=0.5, "RobotDriveDevRef"=w485) -> ("RobotDriveDevRef 2"=w484:T1)  [unwired: 8 in, 1 out]
              n226 = disable-structure shown="Enabled" {
                disable-tunnel: [w528 _] -> w497
                disable-tunnel: w484 -> [w527 _]
                frame Enabled {
                  n227 = disable-structure shown="Enabled" {
                    disable-tunnel: w527 -> [w539 _]
                    disable-tunnel: 1.0 -> [w538 _]
                    disable-tunnel: 0.0 -> [w535 _]
                    disable-tunnel: 0.0 -> [w534 _]
                    disable-tunnel: [w532 _] -> w528
                    frame Enabled {
                      n228 = global read "Robot Global Data.vi" "VComp Enable"() -> (w533:bool)
                      n229 = call "2039_hw MecanumCartesian.vi"("VComp Scaling"=w533, "Rotation"=w538, "Y"=w534, "X"=w535, "RobotDriveDevRef"=w539) -> ("Motor Values"=w536:dbl[], "RobotDriveDevRef"=w532:T1)  [unwired: 4 in, 1 out]
                      n230 = call-poly <vilib>:"NT Write Value.vi"("Numeric Array"=w536, "Name"="Mecanum Drive") -> ()  [unwired: 9 in, 1 out]
                    }
                    frame Disabled {
                    }
                  }
                }
                frame Disabled {
                }
              }
              n231 = call <vilib>:"WPI_RobotDriveDelayAndUpdateSafety.vi"("Delay (s)"=0.65, "RobotDriveDevRef"=w497) -> ("RobotDriveDevRef 2"=w496:T1)  [unwired: 8 in, 1 out]
              n232 = disable-structure shown="Enabled" {
                disable-tunnel: [w515 _] -> w494
                disable-tunnel: w496 -> [w514 _]
                frame Enabled {
                  n233 = disable-structure shown="Enabled" {
                    disable-tunnel: w514 -> [w526 _]
                    disable-tunnel: 0.0 -> [w519 _]
                    disable-tunnel: 0.0 -> [w523 _]
                    disable-tunnel: 0.5 -> [w522 _]
                    disable-tunnel: [w520 _] -> w515
                    frame Enabled {
                      n234 = global read "Robot Global Data.vi" "VComp Enable"() -> (w521:bool)
                      n235 = call "2039_hw MecanumCartesian.vi"("VComp Scaling"=w521, "Rotation"=w519, "Y"=w522, "X"=w523, "RobotDriveDevRef"=w526) -> ("Motor Values"=w524:dbl[], "RobotDriveDevRef"=w520:T1)  [unwired: 4 in, 1 out]
                      n236 = call-poly <vilib>:"NT Write Value.vi"("Numeric Array"=w524, "Name"="Mecanum Drive") -> ()  [unwired: 9 in, 1 out]
                    }
                    frame Disabled {
                    }
                  }
                }
                frame Disabled {
                }
              }
              n237 = call <vilib>:"WPI_RobotDriveDelayAndUpdateSafety.vi"("Delay (s)"=1.25, "RobotDriveDevRef"=w494) -> ()  [unwired: 8 in, 2 out]
            }
          }
          n238 = global write "Robot Global Data.vi" "VComp Enable"(FALSE) -> ()
        }
      }
    }
  }
  n239 = call <vilib>:"WPI_DriverStationGet Alliance Info.vi"() -> ()  [unwired: 12 out]
  n240 = while {
    stop <- FALSE stop-if-true
    n241 = call <vilib>:"WPI_DriverStationReport Robot Code State.vi"("Autonomous"=TRUE) -> ()  [unwired: 10 in, 1 out]
    n242 = Wait (ms)(milliseconds to wait=u32 20) -> ()  [unwired: 1 out]
  }
